vi "R_INIT.vi"(1 "install path":path=path "C:/Program Files (x86)/National Instruments/LabLinda", 2 "Cleneup":bool, 7 "Ip":string, 11 "error in (no error)":errorcluster, 12 "Space size":i32=100000) -> (15 "error out":errorcluster)   [LabVIEW 2015]
doc: "REMOTE OUT"
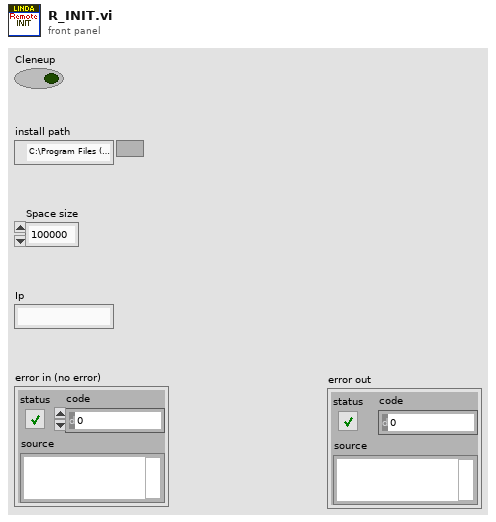
[diagram p1: front panel]
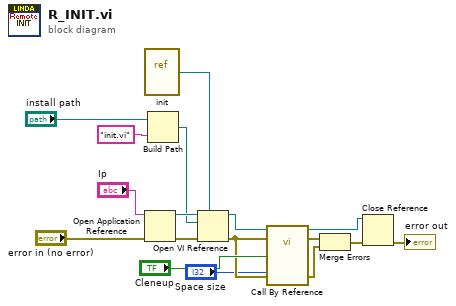
[diagram p0: block diagram]
diagram:
  n1 = vi-ref "init.vi"() -> (w6:refnum<vi>)
  n2 = Open Application Reference(8:"error in (no error)", 11:"Ip") -> (0:w12:errorcluster, 3:w15:refnum<vi>)  [unwired: 2 in]
  n3 = Build Path(base path="install path", name or relative path="init.vi") -> (appended path=w13:path)
  n4 = Open VI Reference(type specifier VI Refnum (for type only)=w6, application reference (local)=w15, vi path=w13, error in (no error)=w12) -> (vi reference=w5:refnum<vi>, error out=w2:errorcluster)  [unwired: 2 in]
  n5 = call-by-ref "?"(reference=w5, error in=w2, "Space size"="Space size", "Cleaneup"="Cleneup", 8:"error in (no error)"=w2) -> (reference out=w9:refnum<vi>, error out=w11:errorcluster, 0:"error out"=w3:errorcluster)  [unwired: 8 in]
  n6 = Merge Errors(w11, w3) -> (w10:errorcluster)
  n7 = Close Reference(reference=w9, error in (no error)=w10) -> (error out=→"error out":errorcluster)
